vi "Test.vi"() -> ()   [LabVIEW 2021]
panel:
  in  "Color Box":u32(colorbox)=65280
  out "appended array":u32[](array[numeric])
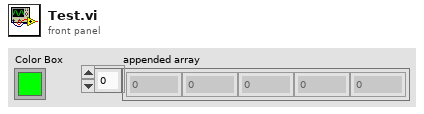
[diagram p1: front panel]
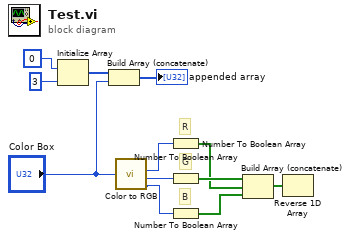
[diagram p0: block diagram]
diagram:
  # "G"
  # "B"
  # "R"
  n1 = Initialize Array(0 ("Color"), 3 ("dimension size")) -> (w12:i32[])
  n2 = Build Array (concatenate)(w12, "Color Box") -> (→"appended array":u32[])
  n3 = call <vilib>:"Color to RGB.vi"("Color"="Color Box") -> ("R"=w5:u8, "G"=w7:u8, "B"=w6:u8)  [unwired: 1 out]
  n4 = Number To Boolean Array(number=w5) -> (Boolean array=w2:bool[])
  n5 = Number To Boolean Array(number=w7) -> (Boolean array=w3:bool[])
  n6 = Number To Boolean Array(number=w6) -> (Boolean array=w1:bool[])
  n7 = Build Array (concatenate)(w3, w2, w1) -> (w4:bool[])
  n8 = Reverse 1D Array(array=w4) -> ()  [unwired: 1 out]
